vi "serialQuery_p.vi"(0 "serialBoard":u16(ring) items=["DEVIL", "M17"], 5 "baseAdderess":u32=3774873600 format="%.0x", 7 "subID1 (0)":u32 format="%.0x", 9 "subID2 (0)":u32, 11 "timeOut [ms] (1000)":i32=1000, 12 "wait [ms] (1000)":i32=1000, 13 "controlCharacter (0)":u16 format="%.0x", 14 "string to write":string) -> (4 "string read":string, 10 "errorCode":cdb format="%.2f", 15 "errorSpec":i32)   [LabVIEW 2010]
doc: "writes the content of the output buffer of the serial port specified by \"subID1\" and \"subID2\", holds on for \"wait\" milliseconds and then get the answer back.\nWARNING: remember to setup the serial channel before running this routine using:\n1. \"serialInitialize.vi\" for hardware setup;\n2. \"serialConfigure\" for software setup."
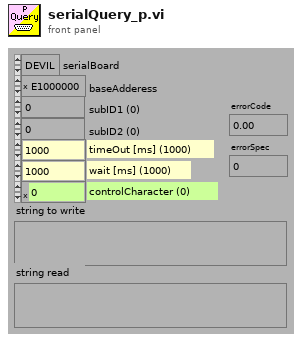
[diagram p1: front panel]
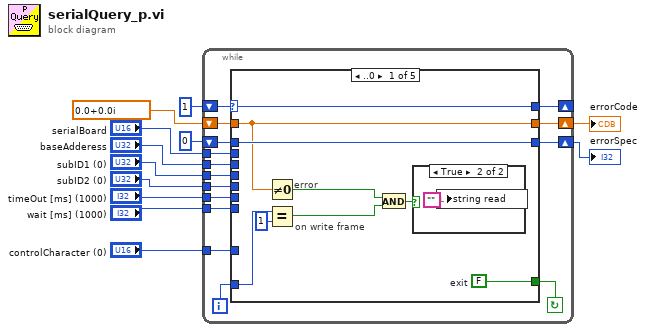
[diagram p0: block diagram]
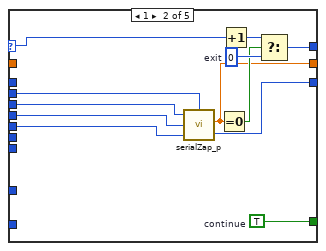
[diagram p3: hidden frame]
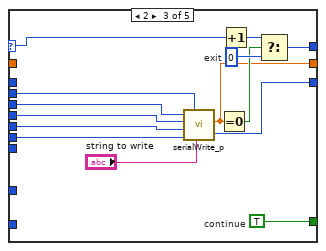
[diagram p4: hidden frame]
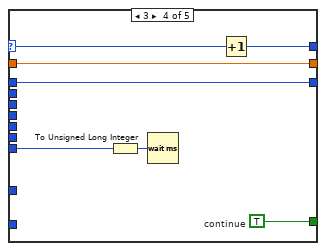
[diagram p5: hidden frame]
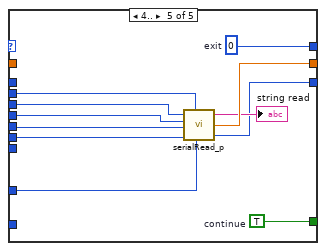
[diagram p6: hidden frame]
diagram:
  n1 = while {
    shift-left: 0 -> [w14]
    shift-right: [w15] -> w2
    tunnel: "wait [ms] (1000)" -> [w16]
    tunnel: "timeOut [ms] (1000)" -> [w17]
    tunnel: "controlCharacter (0)" -> [w18]
    tunnel: "subID2 (0)" -> [w19]
    tunnel: "subID1 (0)" -> [w20]
    tunnel: "baseAdderess" -> [w21]
    tunnel: "serialBoard" -> [w22]
    shift-left: cdb 0.0+0.0i ("errorCode") -> [w26]
    shift-right: [w24] -> w4
    shift-left: 1 -> [w27]
    shift-right: [w25] -> _
    i -> [w13]
    stop <- w23 continue-if-true
    n2 = case shown="..0" w27 {
      selector: w27 -> [w36 w46 w60 w70 _]
      tunnel: w26 -> [w33 _ _ w69 _]
      tunnel: [w36 w47 w61 w68 w72] -> w25
      tunnel: [w33 w44 w58 w69 w80] -> w24
      tunnel: [w35 w43 w57 w67 w79] -> w23
      tunnel: w22 -> [_ w41 w56 _ w78]
      tunnel: w21 -> [_ w40 w55 _ w77]
      tunnel: w20 -> [_ w39 w54 _ w76]
      tunnel: w19 -> [_ w38 w53 _ w75]
      tunnel: w18 -> [_ _ _ _ w74]
      tunnel: w17 -> [_ _ w51 _ w81]
      tunnel: w16 -> [_ _ _ w65 _]
      tunnel: [w34 w42 w52 w64 w71] -> w15
      tunnel: w14 -> [w34 _ _ w64 _]
      tunnel: w13 -> [w30 _ _ _ _]
      frame ..0 {
        w35 = FALSE  # exit
        # "on write frame"
        # "error"
        n3 = Not Equal To 0?(x=w33) -> (x != 0?=w32:bool)
        n4 = Equal?(x=w30, y=1) -> (x = y?=w28:bool)
        n5 = And(x=w32, y=w28) -> (x .and. y?=w31:bool)
        n6 = case shown="True" w31 {
          frame False {
          }
          frame True {
            n7 = local write "string read"("") -> ()
          }
        }
      }
      frame 1 {
        w43 = TRUE  # continue
        w49 = 0  # exit
        n8 = call <userlib>:"serialZap_p.vi"("serialBoard"=w41, "subID2 (0)"=w38, "subID1 (0)"=w39, "baseAdderess"=w40) -> ("errorSpec"=w42:i32, "errorCode"=w44:cdb)
        n9 = Equal To 0?(x=w44) -> (x = 0?=w45:bool)
        n10 = Increment(x=w46) -> (x+1=w48:i32)
        n11 = Select(t=w48, s=w45, f=w49) -> (s? t:f=w47:i32)
      }
      frame 2 {
        w57 = TRUE  # continue
        w63 = 0  # exit
        n12 = call <userlib>:"serialWrite_p.vi"("string to write"="string to write", "serialBoard"=w56, "timeOut [ms] (1000)"=w51, "subID2 (0)"=w53, "subID1 (0)"=w54, "baseAdderess"=w55) -> ("errorSpec"=w52:i32, "errorCode"=w58:cdb)
        n13 = Equal To 0?(x=w58) -> (x = 0?=w59:bool)
        n14 = Increment(x=w60) -> (x+1=w62:i32)
        n15 = Select(t=w62, s=w59, f=w63) -> (s? t:f=w61:i32)
      }
      frame 3 {
        w67 = TRUE  # continue
        n16 = To Unsigned Long Integer(number=w65) -> (unsigned 32bit integer=w66:u32)
        n17 = Wait (ms)(milliseconds to wait=w66) -> ()  [unwired: 1 out]
        n18 = Increment(x=w70) -> (x+1=w68:i32)
      }
      frame 4.. {
        w79 = TRUE  # continue
        w72 = 0  # exit
        n19 = call <userlib>:"serialRead_p.vi"("baseAdderess"=w77, "serialBoard"=w78, "subID1 (0)"=w76, "subID2 (0)"=w75, "controlCharacter (0)"=w74, "timeOut [ms] (1000)"=w81) -> ("string read"=→"string read":string, "errorCode"=w80:cdb, "errorSpec"=w71:i32)
      }
    }
  }
  "errorCode" <- w4
  "errorSpec" <- w2
